vi "Instrument Do Core.vi"(8 "error in (no error)":errorcluster, 9 "Instrument in":refnum<class "Instrument Driver.lvclass">, 10 "Actor in":refnum<class "Actor.lvclass">, 11 "DMM Config Msg in":refnum<class "DMM Config Msg.lvclass">) -> (0 "error out":errorcluster, 1 "Instrument out":refnum<class "Instrument Driver.lvclass">, 2 "Actor out":refnum<class "Actor.lvclass">, 3 "DMM Config Msg out":refnum<class "DMM Config Msg.lvclass">, 5 "Data":refnum<class "Data.lvclass">)   [LabVIEW 2020, in "DMM Msg.lvlib" / "DMM Config Msg.lvclass"]
doc: "Set the configuration on the DMM and return the Success boolean in a generic Boolean class."
uses:
  DMM Config Msg.lvclass
  PPL/HDH.Actor Framework.Core.Actor.lvlibp/1abvi3w/vi.lib/ActorFramework/Actor/Actor.lvclass
  PPL/HDH.Data.Generic.lvlibp/Data.lvclass
  PPL/HDH.Actor Framework.Core.Instrument Driver.lvlibp/Instrument Driver/Instrument Driver.lvclass
  PPL/HDH.Driver.DMM.lvlibp/DMM Driver.lvclass
  C:/Current projects/WS/PPL/HDH.Actor Framework.Core.Instrument Driver.lvlibp/Instrument Driver/Instrument Driver.lvclass
  DMM Config Msg.lvclass/DMM Config Msg.ctl
  PPL/HDH.Data.Generic.lvlibp/Generic Data/Boolean/Boolean.lvclass
  C:/Current projects/WS/PPL/HDH.Data.Generic.lvlibp/Data.lvclass
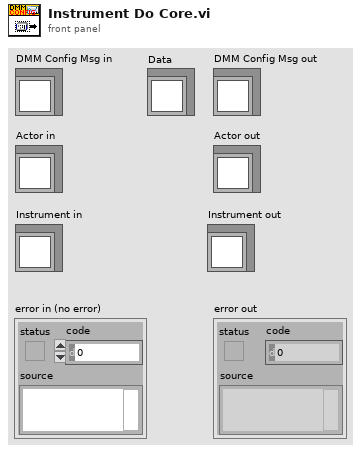
[diagram p1: front panel]
types:
  T1 = typedef "HDH.Driver.DMM.lvlibp/Ctl_Function.ctl" = enum8{"DC Volts", "AC Volts", "DC Current", "AC Current", "2-wire Resistance", "4-wire Resistance", "Diode", "Frequency", "Period", "AC Volts DC Coupled", "Capacitance", "Inductance", "Temperature"}
  T2 = typedef "HDH.Driver.DMM.lvlibp/Ctl_DigitResolution.ctl" = enum8{"3½", "4½", "5½", "6½", "7½"}
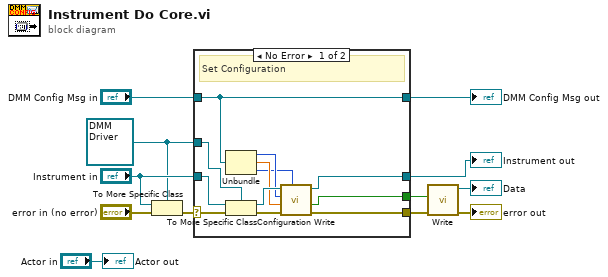
[diagram p0: block diagram]
diagram:
  w5 = refnum<class "DMM Driver.lvclass"> refnum ("HDH.Driver.DMM.lvlibp:DMM Driver.lvclass")
  n1 = To More Specific Class(target class=w5, reference="Instrument in", error in="error in (no error)") -> (error out=w10:errorcluster)  [unwired: 1 out]
  n2 = case shown="No Error" w10 {
    selector: w10 -> [w23 w26]
    tunnel: [w15 w26] -> w1
    tunnel: [w13 w25] -> w9
    tunnel: "DMM Config Msg in" -> [w13 w25]
    tunnel: [w14 w24] -> w7
    tunnel: "Instrument in" -> [w22 w24]
    tunnel: w5 -> [w21 _]
    tunnel: [w12 _] -> w3
    frame No Error {
      # "Set Configuration"
      n3 = Unbundle(w13) -> (w18:T1, w17:dbl, w16:T2)
      n4 = To More Specific Class(target class=w21, reference=w22, error in=w23) -> (specific class reference=w20:refnum<class "DMM Driver.lvclass">, error out=w19:errorcluster)
      n5 = call "Configuration Write.vi"("Digit Resolution(5½)"=w16, "error in (no error)"=w19, "Range"=w17, "Function"=w18, "DMM Driver in"=w20) -> ("error out"=w15:errorcluster, "Success?"=w12:bool, "DMM Driver out"=w14:refnum<class "DMM Driver.lvclass">)  [unwired: 4 in]
    }
    frame Error {
      # "Incorrect instrument - Return error"
    }
  }
  "error out" <- w1
  "DMM Config Msg out" <- w9
  "Instrument out" <- w7
  n6 = call "Write.vi"("Boolean"=w3) -> ("Boolean out"=→"Data":refnum<class "Boolean.lvclass">)  [unwired: 10 in]
  "Actor out" <- "Actor in"
